vi "Read.vi"(8 "error in (no error)":errorcluster caption="entrée d'erreur (pas d'erreur)") -> (0 "error out":errorcluster caption="sortie d'erreur", 3 "Open Out":string)   [LabVIEW 2012, in "TiffLib_v2.lvlib"]
uses:
  TiffLib_v2.lvlib
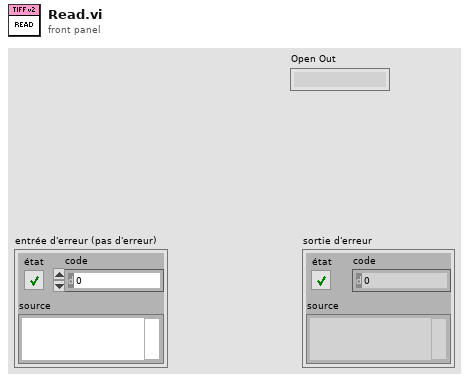
[diagram p1: front panel]
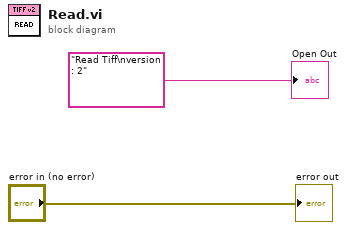
[diagram p0: block diagram]
diagram:
  "error out" <- "error in (no error)"
  "Open Out" <- "Read Tiff\nversion : 2" ("chaîne de format")
